vi "AFM_DLog.LogDataToDataBase.vi"(8 "Set Resistance":T1(ring)=enum."1G ohm", 9 "Litho":T2(array[cluster]), 10 "Name":string, 11 "Instrument.AFM_DLog in":refnum<class "Instrument.AFM_DLog.lvclass">) -> (3 "Instrument.AFM_DLog out":refnum<class "Instrument.AFM_DLog.lvclass">)   [LabVIEW 2019, in "Instrument.AFM_DLog.lvclass"]
uses:
  Instrument.AFM_DLog.lvclass
  C:/Program Files/National Instruments/LabVIEW 2019/user.lib/Levylab/Instrument Framework/Instrument/Instrument.lvclass
  d0e9106d-912d-4541-b628-30ffe06d549f.vi
  <vilib>/Utility/Data Type/Get Type Information.vi
  <vilib>/Utility/Data Type/Get Numeric Information.vi
  <userlib>/_OpenG.lib/lvdata/lvdata.llb/Unwrap VVariant__ogtk.vi
  <userlib>/Levylab/Instrument Framework/Instrument/Instrument.lvclass
  C:/Program Files/National Instruments/LabVIEW 2019/user.lib/LevyLab/Instrument Framework/Instrument Types/SCPI/Instrument.SCPI.lvclass
  C:/Program Files/National Instruments/LabVIEW 2019/vi.lib/JKI/JKI SMO/SMO/SMO.lvclass
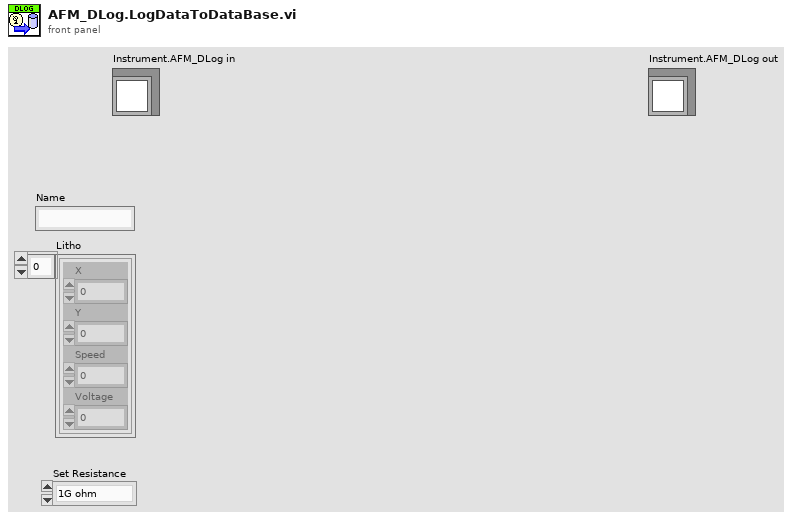
[diagram p1: front panel]
types:
  T1 = enum16{"open", "discharge tip", "0 ohms", "100k ohm", "10M ohm", "1G ohm"}
  T2 = cluster{"X":dbl, "Y":dbl, "Speed":dbl, "Voltage":dbl}[]
  T3 = cluster{"Litho[0]":cluster{"X":dbl, "Y":dbl, "Speed":dbl, "Voltage":dbl}, "Litho[1]":cluster{"X":dbl, "Y":dbl, "Speed":dbl, "Voltage":dbl}, "Litho[2]":cluster{"X":dbl, "Y":dbl, "Speed":dbl, "Voltage":dbl}, "Litho[3]":cluster{"X":dbl, "Y":dbl, "Speed":dbl, "Voltage":dbl}, "Litho[4]":cluster{"X":dbl, "Y":dbl, "Speed":dbl, "Voltage":dbl}, "Litho[5]":cluster{"X":dbl, "Y":dbl, "Speed":dbl, "Voltage":dbl}, "Litho[6]":cluster{"X":dbl, "Y":dbl, "Speed":dbl, "Voltage":dbl}, "Litho[7]":cluster{"X":dbl, "Y":dbl, "Speed":dbl, "Voltage":dbl}, "Litho[8]":cluster{"X":dbl, "Y":dbl, "Speed":dbl, "Voltage":dbl}}
  T4 = cluster{"Name":string, "Speed":dbl, "Voltage":dbl, "string out":string}
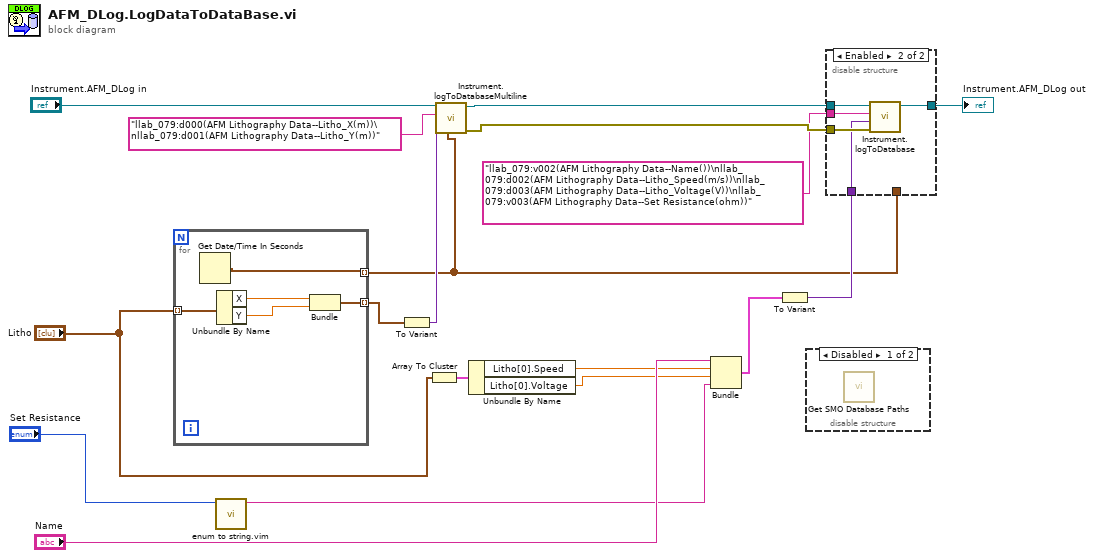
[diagram p0: block diagram]
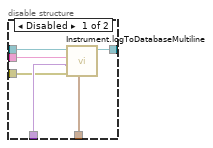
[diagram p2: hidden frame]
diagram:
  n1 = for {
    tunnel: "Litho" -> [w23] mode=indexing
    tunnel: [w22] -> w18 mode=indexing
    tunnel: [w19] -> w2 mode=indexing
    n2 = Get Date/Time In Seconds() -> (seconds since 1Jan1904=w19:timestamp)
    n3 = Unbundle By Name(w23) -> ("X"=w21:dbl, "Y"=w20:dbl)
    n4 = Bundle("X"=w21, "Y"=w20) -> (w22:cluster{"X":dbl, "Y":dbl})  [unwired: 1 in]
  }
  n5 = call "enum to string.vim"("enum in"="Set Resistance") -> ("string out"=w11:string)  [unwired: 9 in, 1 out]
  n6 = To Variant(anything=w18) -> (Variant=w8:variant)
  n7 = Array To Cluster(array="Litho") -> (cluster=w15:T3)
  n8 = call <userlib>:"Instrument.logToDatabaseMultiline.vi"("timestamps"=w2, "Data"=w8, "Paths"="llab_079:d000(AFM Lithography Data--Litho_X(m))\nllab_079:d001(AFM Lithography Data--Litho_Y(m))", "Instrument"="Instrument.AFM_DLog in") -> ("error out"=w3:errorcluster, "Instrument out"=w6:refnum<class "Instrument.AFM_DLog.lvclass">)  [unwired: 6 in]
  n9 = Unbundle By Name(w15) -> ("Litho[0].Speed"=w13:dbl, "Litho[0].Voltage"=w12:dbl)
  n10 = Bundle("Name"="Name", "Speed"=w13, "Voltage"=w12, "string out"=w11) -> (w10:T4)  [unwired: 1 in]
  n11 = To Variant(anything=w10) -> (Variant=w4:variant)
  n12 = disable-structure shown="Disabled" {
    frame Disabled {
      n13 = call-dynamic "Get SMO Database Paths.vi"() -> ()  [unwired: 9 in, 3 out]
    }
    frame Enabled {
    }
  }
  n14 = disable-structure shown="Enabled" {
    disable-tunnel: w6 -> [w29 w33]
    disable-tunnel: [w28 w34] -> w5
    disable-tunnel: "llab_079:v002(AFM Lithography Data--Name())\nllab_079:d002(AFM Lithography Data--Litho_Speed(m/s))\nllab_079:d003(AFM Lithography Data--Litho_Voltage(V))\nllab_079:v003(AFM Lithography Data--Set Resistance(ohm))" ("Paths") -> [w27 w32]
    disable-tunnel: w4 -> [w26 w30]
    disable-tunnel: w3 -> [w25 w31]
    disable-tunnel: w2 -> [w24 _]
    frame Disabled {
      n15 = call <userlib>:"Instrument.logToDatabaseMultiline.vi"("timestamps"=w24, "error in (no error)"=w25, "Data"=w26, "Paths"=w27, "Instrument"=w29) -> ("Instrument out"=w28:refnum<class "Instrument.AFM_DLog.lvclass">)  [unwired: 5 in, 1 out]
    }
    frame Enabled {
      n16 = call <userlib>:"Instrument.logToDatabase.vi"("error in (no error)"=w31, "Data"=w30, "Paths"=w32, "Instrument"=w33) -> ("Instrument out"=w34:refnum<class "Instrument.AFM_DLog.lvclass">)  [unwired: 6 in, 1 out]
    }
  }
  "Instrument.AFM_DLog out" <- w5
